vi "sub UI check value valid.vi"(8 "error in":errorcluster, 11 "num ref":refnum<vi>) -> (0 "error out":errorcluster, 3 "valid":bool)   [LabVIEW 2018, in "LF2R IDE.lvlib" / "LF2R IDE.lvclass"]
uses:
  LF2R IDE.lvclass
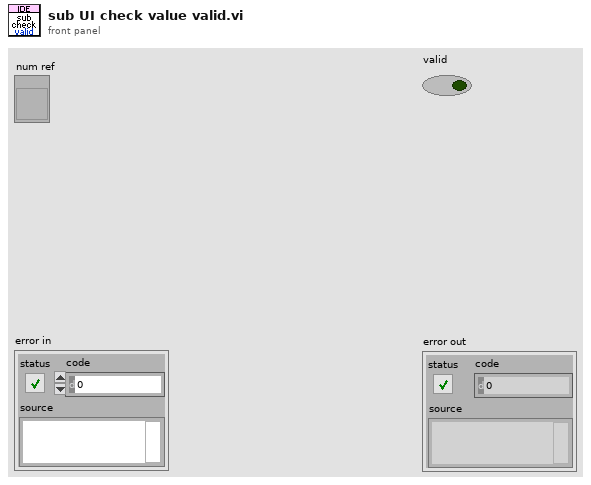
[diagram p1: front panel]
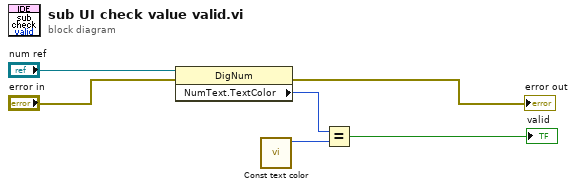
[diagram p0: block diagram]
diagram:
  n1 = property class="DigNum"(reference="num ref", error in="error in") -> (error out=→"error out":errorcluster, "NumText.TextColor"=w3:u32)  [unwired: 1 out]
  n2 = call "Const text color.vi"() -> ("valid num color"=w2:u32)  [unwired: 10 in, 1 out]
  n3 = Equal?(x=w3, y=w2) -> (x = y?=→"valid":bool)
